vi "Color Interpolate T4 T5.vi"(0 "a_data":dbl[](array[numeric]), 1 "a_zarray":dbl[](array[numeric]), 5 "a_NumPoints":u16, 7 "a_Observer":u8, 9 "a_xarray":dbl[](array[numeric]), 11 "a_yarray":dbl[](array[numeric]), 12 "error in (no error)":errorcluster) -> (4 "a_data out":dbl[](array[numeric]), 6 "function return":i16, 8 "a_xarray out":dbl[](array[numeric]), 10 "a_yarray out":dbl[](array[numeric]), 14 "error out":errorcluster, 15 "a_zarray out":dbl[](array[numeric]))   [LabVIEW 2013, in "AVSirrad.lvlib"]
doc: "DLL_API short int __stdcall Color_GetColorRenderingIndex\n(\n DataType *a_data,\n unsigned char a_CIEResolution,\n unsigned char a_Observer,\n double *R_Values,\n double *CRI\n);"
uses:
  AVSirrad.lvlib
  AVSIRRAD/Examples/Labview/build/AVSirrad.dll
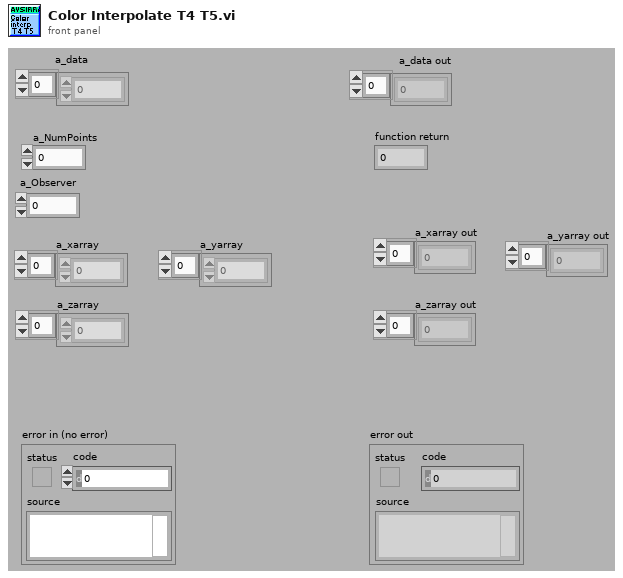
[diagram p1: front panel]
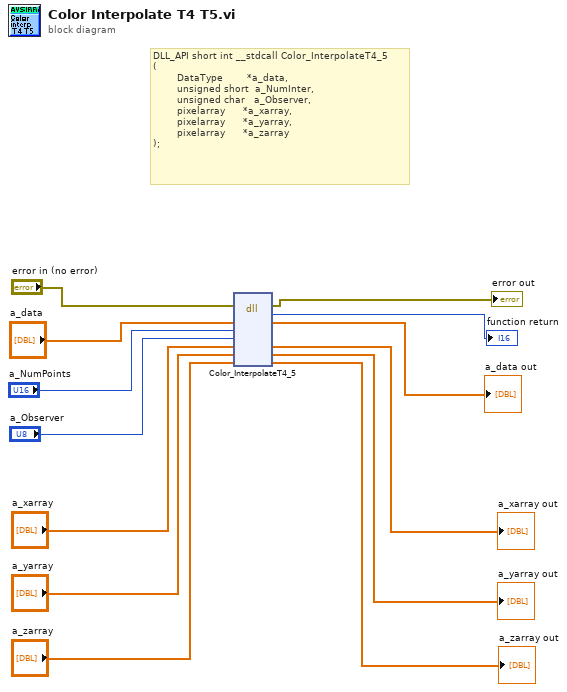
[diagram p0: block diagram]
diagram:
  # "DLL_API short int __stdcall Color_InterpolateT4_5\n(\n        DataType        *a_data,\n        unsigned short  a_NumInter,\n        unsigned char   a_Observer,\n        pixelarray      *a_xarray,\n        pixelarray      *a_yarray,\n        pixelarray      *a_zarray\n);"
  n1 = dll-call lib="C:/AVSIRRAD/Examples/Labview/build/AVSirrad.*" fn="Color_InterpolateT4_5"(error in="error in (no error)", "a_data"="a_data", "a_NumInter"="a_NumPoints", "a_Observer"="a_Observer", "a_xarray"="a_xarray", "a_yarray"="a_yarray", "a_zarray"="a_zarray") -> (error out=→"error out":errorcluster, "return type"=→"function return":i16, "a_data"=→"a_data out":dbl[], "a_xarray"=→"a_xarray out":dbl[], "a_yarray"=→"a_yarray out":dbl[], "a_zarray"=→"a_zarray out":dbl[])  [unwired: 4 in, 1 out]
